vi "ParseString.vi"(1 "Input String":string, 4 "Classifier":string) -> (17 "Output Array":dbl[][](graph))   [LabVIEW 2022 SP3]
panel:
  out "Parsing Result":string
  out "Input class":string
  out "Output String":string
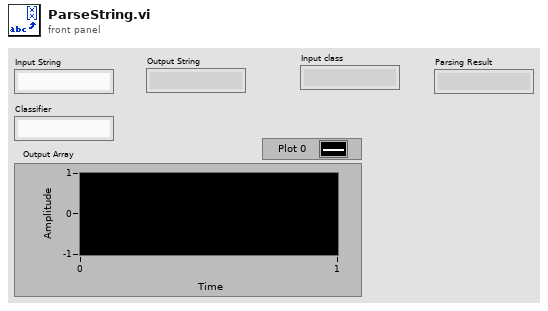
[diagram p1: front panel]
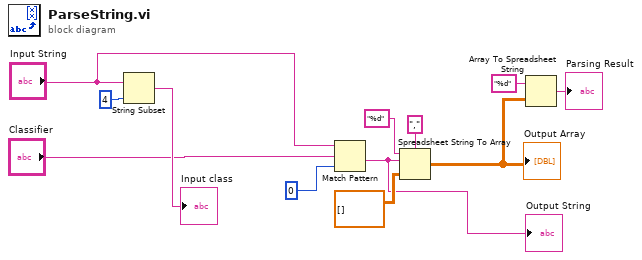
[diagram p0: block diagram]
diagram:
  n1 = String Subset(string="Input String", length (rest)=4 ("length (rest)")) -> (substring=→"Input class":string)  [unwired: 1 in]
  n2 = Match Pattern(string="Input String", regular expression="Classifier", offset (0)=0) -> (after substring=w4:string)  [unwired: 3 out]
  "Output String" <- w4
  n3 = Spreadsheet String To Array(delimiter (Tab)=",", format string="%d", spreadsheet string=w4, array type (2D Dbl)=dbl[][] []) -> (array=w5:dbl[][])
  "Output Array" <- w5
  n4 = Array To Spreadsheet String(array=w5, 3:"%d" ("format string")) -> (spreadsheet string=→"Parsing Result":string)  [unwired: 1 in]
